vi "write_node_object_dictionary.vi"(8 "num":u64, 9 "subind":u8, 10 "index":u16, 11 "node":u8) -> (2 "num":u64, 3 "return":i16)   [LabVIEW 2011]
uses:
  canopen_dll_master.dll
panel:
  in  "num":cluster{"num":u64}
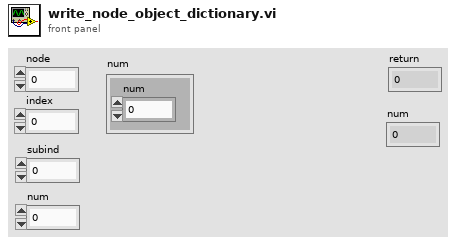
[diagram p1: front panel]
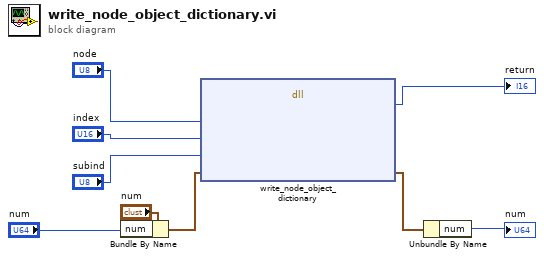
[diagram p0: block diagram]
diagram:
  n1 = Bundle By Name(cluster="num", "num"="num") -> (w3:cluster{"num":u64})
  n2 = dll-call lib="canopen_dll_master.dll" fn="write_node_object_dictionary"("node"="node", "index"="index", "subind"="subind", "num"=w3) -> ("return type"=→"return":i16, "num"=w1:cluster{"num":u64})  [unwired: 6 in, 2 out]
  n3 = Unbundle By Name(w1) -> ("num"=→"num":u64)
